vi "Finalize To Settings.vi"(8 "error in (no error)":errorcluster, 11 "Thread Configuration in":refnum<class "Thread Configuration.lvclass">) -> (0 "error out":errorcluster, 2 "settings":cluster{"key":string, "value":string}[](array[cluster]), 3 "Thread Configuration out":refnum<class "Thread Configuration.lvclass">)   [LabVIEW 2017, in "GE Reflective Memory.lvlib" / "Thread Configuration.lvclass"]
uses:
  Thread Configuration.lvclass
  Thread Configuration.lvclass/Thread Configuration.ctl
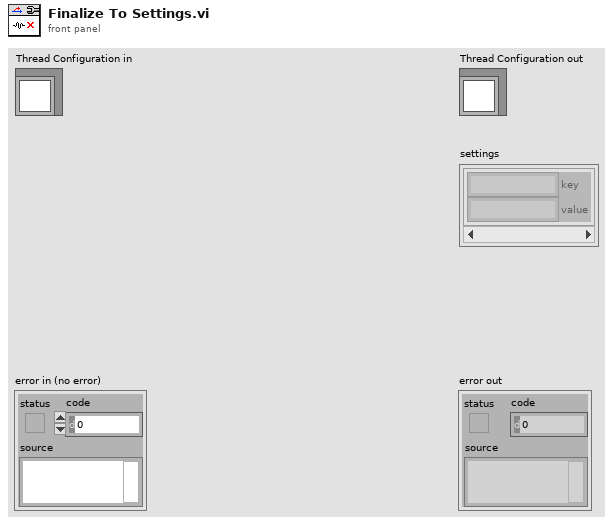
[diagram p1: front panel]
types:
  T1 = typedef "GE 5565PIORC.lvclass/GE 5565PIORC.Typedef.DMA Wait Mode.ctl" = enum16{"Polling", "Interrupt"}
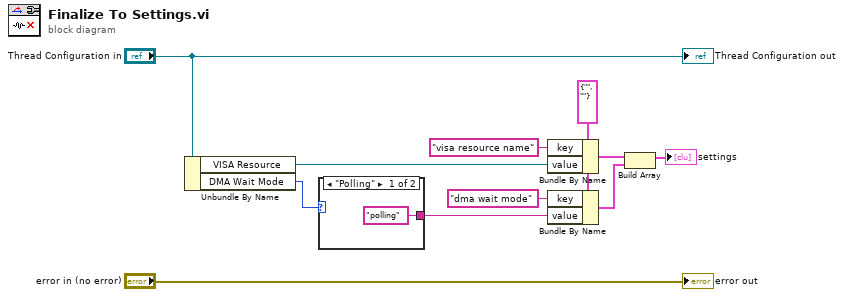
[diagram p0: block diagram]
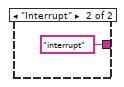
[diagram p2: hidden frame]
diagram:
  w7 = cluster{"key":string, "value":string} {"key"="", "value"=""} ("setting")
  n1 = Unbundle By Name("Thread Configuration in") -> ("VISA Resource"=w3:refnum<visa-resource-name>, "DMA Wait Mode"=w6:T1)
  n2 = case shown="\"Polling\"" w6 {
    tunnel: ["polling" ("y") "interrupt" ("y")] -> w5
    frame "Polling" {
    }
    frame "Interrupt" {
    }
  }
  n3 = Bundle By Name(cluster=w7, "key"="visa resource name", "value"=w3) -> (w9:cluster{"key":string, "value":string})
  n4 = Bundle By Name(cluster=w7, "key"="dma wait mode", "value"=w5) -> (w1:cluster{"key":string, "value":string})
  n5 = Build Array(w9, w1) -> (→"settings":cluster{"key":string, "value":string}[])
  "error out" <- "error in (no error)"
  "Thread Configuration out" <- "Thread Configuration in"
